vi "Create TDMS File.vi"(8 "error in (no error)":errorcluster caption="错误输入（无错误）", 11 "Timestamp":timestamp caption="时间标识") -> (0 "error out":errorcluster caption="错误输出", 3 "TDMS File Reference":refnum<k34> caption="TDMS文件引用")   [LabVIEW 2015]
doc: "读取DMA FIFO的波形数据。"
uses:
  Globals/Global - Configuration Options.vi
  Globals/Global - Device Tree Items.vi
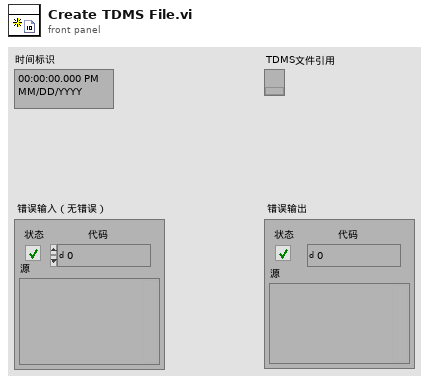
[diagram p1: front panel]
types:
  T1 = enum16{"open", "open or create", "create or replace", "create", "open (read-only)"}
  T2 = cluster{"Left Cell String":string, "Child Text":string[], "Child Tag":string, "Item Indent":i32, "Child Only?":bool, "Glyph Index":i32}[]
  T3 = cluster{"Left Cell String":string, "Child Text":string[], "Child Tag":string, "Item Indent":i32, "Child Only?":bool, "Glyph Index":i32}
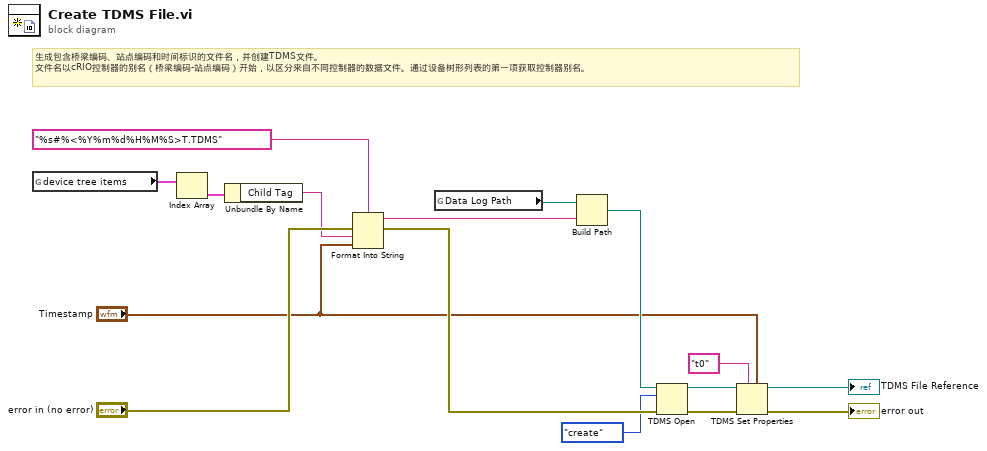
[diagram p0: block diagram]
diagram:
  # "生成包含桥梁编码、站点编码和时间标识的文件名，并创建TDMS文件。\n文件名以cRIO控制器的别名（桥梁编码-站点编码）开始，以区分来自不同控制器的数据文件。通过设备树形列表的第一项获取控制器别名。"
  n1 = global read "Global - Device Tree Items.vi" "device tree items"() -> (w3:T2)
  n2 = Index Array(array=w3) -> (element=w2:T3)  [unwired: 1 in]
  n3 = Unbundle By Name(w2) -> ("Child Tag"=w1:string)
  n4 = Format Into String(format string="%s#%<%Y%m%d%H%M%S>T.TDMS" ("格式字符串"), error in="error in (no error)", w1, "Timestamp") -> (resulting string=w13:string, error out=w15:errorcluster)  [unwired: 1 in]
  n5 = global read "Global - Configuration Options.vi" "Data Log Path"() -> (w12:path)
  n6 = Build Path(base path=w12, name or relative path=w13) -> (appended path=w11:path)
  n7 = TDMS Open(8:w15, 10:T1."create" ("操作(0:open)"), 11:w11) -> (0:w8:errorcluster, 3:w7:refnum<k34>)  [unwired: 4 in]
  n8 = TDMS Set Properties(5:"Timestamp", 7:"t0", 8:w8, 11:w7) -> (0:→"error out":errorcluster, 3:→"TDMS File Reference":refnum<k34>)  [unwired: 2 in, 2 out]
